vi "Wait for Trigger State_Next State Decision.vi"(10 "Acq Hold=0?":bool=TRUE, 11 "Reference Trigger":bool=TRUE) -> (3 "Next State":T1=enum."Arm Acquisition Engine")   [LabVIEW 2012]
uses:
  Acquisition Engine State.ctl
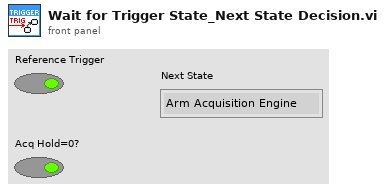
[diagram p1: front panel]
types:
  T1 = typedef "Acquisition Engine State.ctl" = enum8{"Idle", "Arm Acquisition Engine", "Acquire Pre-Trigger Samples", "Wait for Trigger", "Acquisition Hold Off Time", "Read Data from Buffer", "Check Records Done?", "Re-Arm State", "Flush Available Data"}
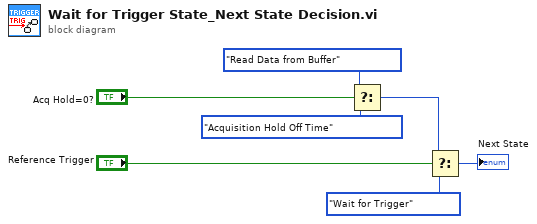
[diagram p0: block diagram]
diagram:
  n1 = Select(t=Acquisition_Engine_State."Read Data from Buffer" ("Acquisition Engine State"), s="Acq Hold=0?", f=Acquisition_Engine_State."Acquisition Hold Off Time") -> (s? t:f=w4:T1)
  n2 = Select(t=w4, s="Reference Trigger", f=Acquisition_Engine_State."Wait for Trigger") -> (s? t:f=→"Next State":T1)
